vi "Create_Time_Vector.vi"(1 "Samping Frequency [Hz]":dbl, 2 "Data Vector [V]":dbl[](array[numeric])) -> (0 "Waveform":waveform(dbl))   [LabVIEW 2023]
doc: "Simple VI to create a Waveform Structure from an input vector and the sampling Frequency, useful to plot time series\nInputs:\n- Array of the signal\n- Sampling Freqency of the aquired signal\nOutputs:\n- Waveform"
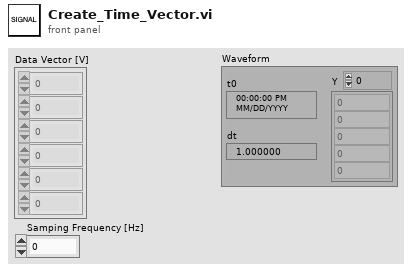
[diagram p1: front panel]
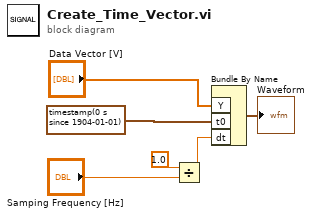
[diagram p0: block diagram]
diagram:
  n1 = Divide(x=1.0, y="Samping Frequency [Hz]") -> (x/y=w3:dbl)
  n2 = Bundle By Name("Y"="Data Vector [V]", "t0"=timestamp(0 s since 1904-01-01), "dt"=w3) -> (→"Waveform":waveform(dbl))  [unwired: 1 in]
